vi "IO4 Interrupt Example.vi"() -> ()   [LabVIEW 2011]
doc: "This example demonstrates the usage of interrupt based IO handling with a IO4 Bricklet. For further explanations see comments on the block diagram."
uses:
  Classes/IO-4 Bricklet/Properties/Read Interrupt.vi
  Classes/IP Connection/IP Connection.lvclass
  Classes/IO-4 Bricklet/IO-4 Bricklet.lvclass
panel:
  out "IO4 States":bool[](array[boolean])
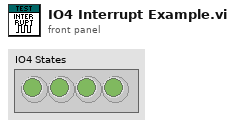
[diagram p1: front panel]
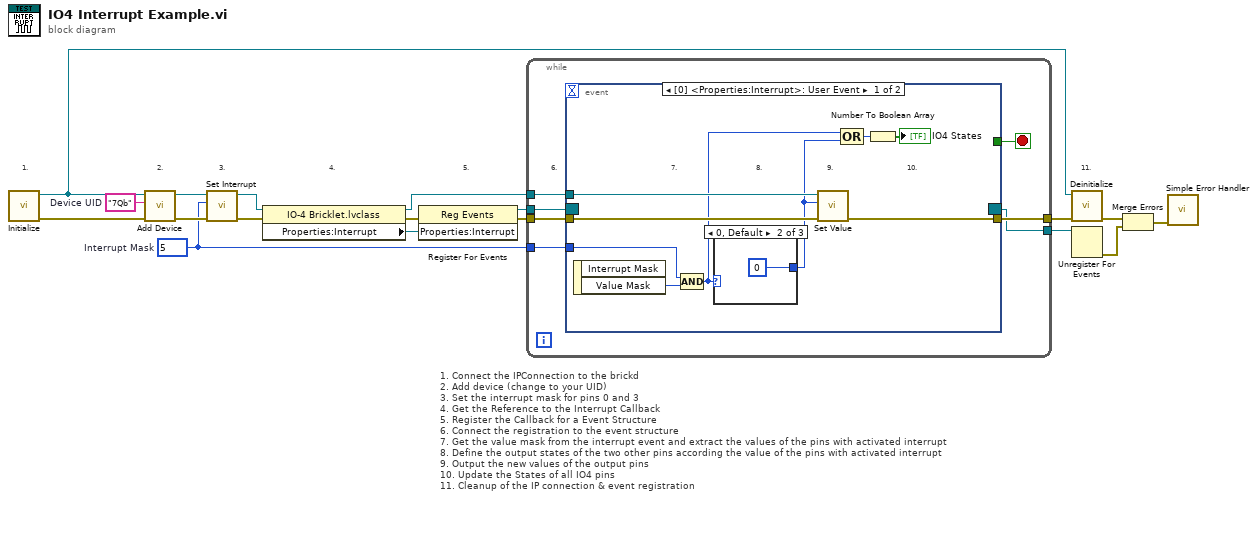
[diagram p0: block diagram]
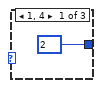
[diagram p2: hidden frame]
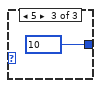
[diagram p3: hidden frame]
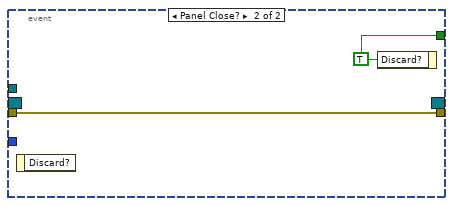
[diagram p4: hidden frame]
diagram:
  w7 = u8 5  # Interrupt Mask
  w18 = "7Qb"  # Device UID
  # "11."
  # "1. Connect the IPConnection to the brickd\n2. Add device (change to your UID)\n3. Set the interrupt mask for pins 0 and 3\n4. Get the Reference to the Interrupt Callback\n5. Register the Callback for a Event Structure\n6. Connect the registration to the event structure\n7. Get the value mask from the interrupt event and extract the values of the pins with activated interrupt\n8. Define the output states of the two other pins according the value of the pins with activated interrupt\n9. Output the new values of the output pins\n10. Update the States of all IO4 pins\n11. Cleanup of the IP connection & event registration"
  # "5."
  # "4."
  # "3."
  # "2."
  # "1."
  n1 = call "Initialize.vi"() -> ("error out"=w17:errorcluster, "IP Connection out"=w6:refnum<class "IP Connection.lvclass">)  [unwired: 10 in]
  n2 = call "Add Device.vi"("Error In"=w17, "Device UID"=w18, "IP Connection"=w6) -> ("Error Out"=w12:errorcluster, "IO-4 Bricklet"=w11:refnum<class "IO-4 Bricklet.lvclass">)  [unwired: 7 in]
  n3 = call "Set Interrupt.vi"("error in (no error)"=w12, "Interrupt Mask"=w7, "IO-4 Bricklet in"=w11) -> ("error out"=w10:errorcluster, "IO-4 Bricklet out"=w9:refnum<class "IO-4 Bricklet.lvclass">)  [unwired: 7 in]
  n4 = property class="IO-4 Bricklet.lvclass"(reference=w9, error in=w10) -> (reference out=w8:refnum<class "IO-4 Bricklet.lvclass">, error out=w16:errorcluster, "Properties:Interrupt"=w15:refnum<user-event>)
  n5 = register-events(error in=w16, w15) -> (reference out=w13:refnum<event-registration>, error out=w14:errorcluster)  [unwired: 1 in]
  n6 = while {
    tunnel: w14 -> [w25]
    tunnel: w13 -> [w24]
    tunnel: w8 -> [w23]
    tunnel: w7 -> [w22]
    tunnel: [w20] -> w5
    tunnel: [w19] -> w3
    stop <- w21 stop-if-true
    # "6."
    n7 = event shown="[0] <Properties:Interrupt>: User Event" {
      selector: w24 -> [_ _]
      dyn-events: [_ _] -> w19
      timeout: _ -> [_ _]
      tunnel: w25 -> [w32 w39]
      tunnel: w23 -> [w31 _]
      tunnel: w22 -> [w33 _]
      tunnel: [w30 w39] -> w20
      tunnel: [_ w38] -> w21
      event User Event {
        # "10."
        # "9."
        # "8."
        # "7."
        n8 = event-data() -> ("Value Mask"=w34:u8)  [unwired: 1 in, 1 out]
        n9 = Compound Arithmetic op=AND(w33, w34) -> (w29:u8)
        n10 = case shown="0, Default" w29 {
          tunnel: [u8 2 ("value") u8 0 ("value") u8 10 ("value")] -> w28
          frame 1, 4 {
          }
          frame 0, Default {
          }
          frame 5 {
          }
        }
        n11 = call "Set Value.vi"("error in (no error)"=w32, "Value Mask"=w28, "IO-4 Bricklet in"=w31) -> ("error out"=w30:errorcluster)  [unwired: 7 in, 1 out]
        n12 = Compound Arithmetic op=OR(w29, w28) -> (w27:u8)
        n13 = Number To Boolean Array(number=w27) -> (Boolean array=→"IO4 States":bool[])
      }
      event Panel Close? {
        w38 = TRUE ("Discard?")
        n14 = event-data() -> ()  [unwired: 1 in, 1 out]
        n15 = event-data("Discard?"=w38) -> ()  [unwired: 1 in, 1 out]
      }
    }
  }
  n16 = call "Deinitialize.vi"("error in (no error)"=w5, "IP Connection in"=w6) -> ("error out"=w4:errorcluster)  [unwired: 9 in]
  n17 = Unregister For Events(event registration refnum=w3) -> (error out=w1:errorcluster)  [unwired: 1 in]
  n18 = Merge Errors(w4, w1) -> (w2:errorcluster)
  n19 = call <vilib>:"Simple Error Handler.vi"("error in (no error)"=w2) -> ()  [unwired: 4 in, 5 out]
